vi "Find 2601B.vi"(8 "错误输入（无错误）":errorcluster) -> (0 "错误输出":errorcluster, 3 "VISA资源名称输出":refnum<visa-resource-name>, 5 "仪器存在":bool)   [LabVIEW 2021]
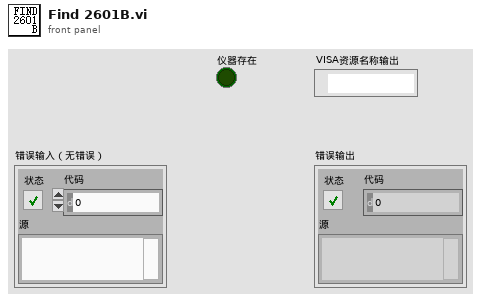
[diagram p1: front panel]
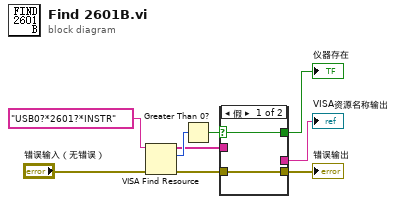
[diagram p0: block diagram]
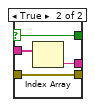
[diagram p2: hidden frame]
diagram:
  n1 = VISA Find Resource(8:"错误输入（无错误）", 11:"USB0?*2601?*INSTR" ("表达式(\"?*\")")) -> (0:w4:errorcluster, 2:w7:u32, 3:w3:string[])  [unwired: 1 in]
  n2 = Greater Than 0?(x=w7) -> (x > 0?=w6:bool)
  n3 = case shown="假" w6 {
    selector: w6 -> [w11 w12]
    tunnel: [w10 w15] -> w5
    tunnel: w4 -> [w10 w15]
    tunnel: w3 -> [_ w14]
    tunnel: [_ w13] -> w2
    tunnel: [w11 w12] -> w1
    frame False {
    }
    frame True {
      n4 = Index Array(array=w14) -> (element=w13:string)  [unwired: 1 in]
    }
  }
  "仪器存在" <- w1
  "VISA资源名称输出" <- w2
  "错误输出" <- w5
